vi "Host - Thruster Cmd encode Serial (SubVI).vi"(11 "Serial":string[][](array[string])) -> (3 "Serial Data":T1[](array[typedef]))   [LabVIEW 2021]
uses:
  Async Serial/Controls/Async Update Cluster.ctl
  Async Serial/Controls/Async Message Info Cluster.ctl
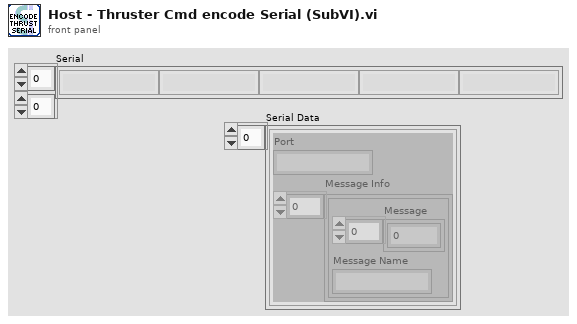
[diagram p1: front panel]
types:
  T1 = typedef "Async Update Cluster.ctl" = cluster{"Port":string, "Message Info":T2[]}
  T2 = typedef "Async Message Info Cluster.ctl" = cluster{"Message":u8[], "Message Name":string}
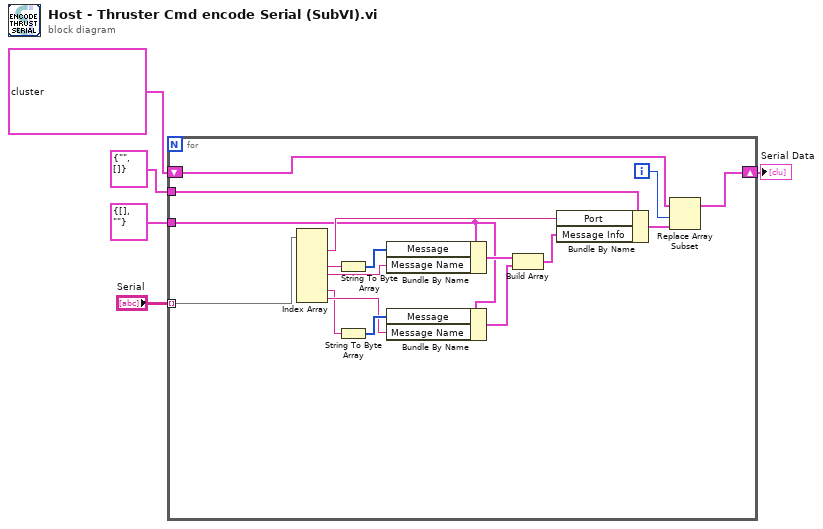
[diagram p0: block diagram]
diagram:
  n1 = for {
    shift-right: [w21] -> w2
    shift-left: T1[] [{"Port"="", "Message Info"=[{"Message"=[0], "Message Name"=""}, {"Message"=[0], "Message Name"=""}]}] ("Serial Data") -> [w22]
    tunnel: "Serial" -> [w18] mode=indexing
    tunnel: T1 {"Port"="", "Message Info"=[]} ("new element/subarray") -> [w19]
    tunnel: T2 {"Message"=[], "Message Name"=""} ("Message Info") -> [w8]
    i -> [w20]
    n2 = Index Array(array=w18) -> (element #1=w17:string, element #3=w13:string, element #4=w12:string, element #6=w6:string, element #7=w7:string)  [unwired: 7 in, 2 out]
    n3 = String To Byte Array(string=w13) -> (unsigned byte array=w16:u8[])
    n4 = String To Byte Array(string=w6) -> (unsigned byte array=w10:u8[])
    n5 = Bundle By Name(cluster=w8, "Message"=w16, "Message Name"=w12) -> (w15:T2)
    n6 = Bundle By Name(cluster=w8, "Message"=w10, "Message Name"=w7) -> (w9:T2)
    n7 = Build Array(w15, w9) -> (w14:T2[])
    n8 = Bundle By Name(cluster=w19, "Port"=w17, "Message Info"=w14) -> (w11:T1)
    n9 = Replace Array Subset(array=w22, new element=w11, index=w20) -> (w21:T1[])
  }
  "Serial Data" <- w2
